vi "Begin.vi"(11 "Image Size":T1=enum."160x120") -> (0 "error out":errorcluster)   [LabVIEW 2012]
doc: "Called before other user functions, this VI is expected to open initial I/O refnums, load in file data, and do all program initialization. Notice that the <B>error out</B> terminal is simply used for data flow. Wiring it to other structures or subVIs ensures that this VI runs first."
uses:
  <vilib>/Rock Robotics/WPI/Camera/WPI_CameraImageSize.ctl
  <vilib>/Rock Robotics/WPI/DriverStation/WPI_DriverStationRobotMode2.ctl
  <vilib>/Rock Robotics/WPI/Joystick/WPI_JoystickDeviceEnum.ctl
  <vilib>/Rock Robotics/WPI/CAN/Jaguar/SubVIs/WPI_CANJaguar_ControlMode.ctl
  <vilib>/Rock Robotics/WPI/CAN/Jaguar/SubVIs/WPI_CANJaguar_SpeedReference.ctl
  <vilib>/Rock Robotics/WPI/CAN/Jaguar/SubVIs/WPI_CANJaguar_BrakeCoastMode.ctl
  <vilib>/Rock Robotics/WPI/CAN/Jaguar/SubVIs/WPI_CANJaguar_PositionReference.ctl
  <vilib>/Rock Robotics/SystemInterfaces/Typedef/FPGA_TypedefDigitalModule.ctl
  <vilib>/Rock Robotics/SystemInterfaces/DIO/FPGA_DIOChannel.ctl
  <vilib>/Rock Robotics/SystemInterfaces/DIO/FPGA_DIORelayChannel.ctl
  <vilib>/Rock Robotics/SystemInterfaces/Typedef/FPGA_TypedefSolenoidModule.ctl
  <vilib>/Rock Robotics/WPI/Solenoid/WPI_SolenoidChannel.ctl
  Robot Global Data.vi
  <vilib>/Rock Robotics/WPI/MotorControl/WPI_MotorControlOpenCANJaguar.vi
  <vilib>/Rock Robotics/WPI/Solenoid/WPI_SolenoidOpenSingle.vi
  <vilib>/Rock Robotics/WPI/Compressor/WPI_CompressorGetSetRefNum.vi
  <vilib>/Rock Robotics/WPI/Camera/WPI_CameraWhite Balance Values.ctl
  <vilib>/Rock Robotics/WPI/Camera/WPI_CameraExposure Values.ctl
  <vilib>/Rock Robotics/WPI/Camera/WPI_CameraFrameRate.ctl
  <vilib>/Rock Robotics/WPI/RobotDrive/WPI_RobotDriveOpen4MotorWithCANJaguar.vi
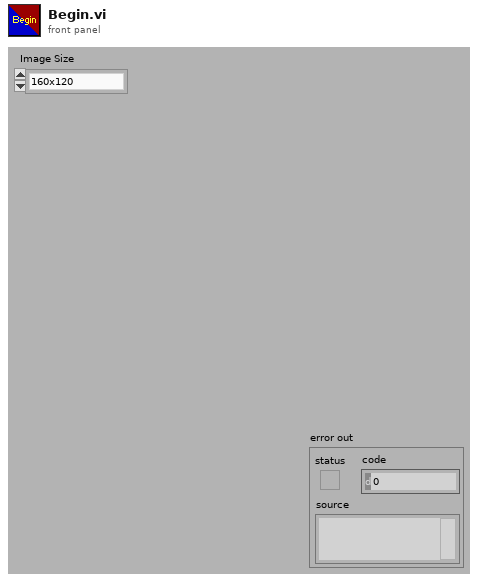
[diagram p1: front panel]
types:
  T1 = typedef "WPI_CameraImageSize.ctl" = enum16{"640x480", "320x240", "160x120"}
  T2 = typedef "WPI_SolenoidChannel.ctl" = enum8{"Solenoid 1", "Solenoid 2", "Solenoid 3", "Solenoid 4", "Solenoid 5", "Solenoid 6", "Solenoid 7", "Solenoid 8", "Invalid"}
  T3 = typedef "FPGA_TypedefSolenoidModule.ctl" = enum16{"Solenoid Module 1", "Solenoid Module 2"}
  T4 = typedef "FPGA_DIORelayChannel.ctl" = enum8{"Relay 1", "Relay 2", "Relay 3", "Relay 4", "Relay 5", "Relay 6", "Relay 7", "Relay 8", "Invalid"}
  T5 = typedef "FPGA_DIOChannel.ctl" = enum8{"DIO 1", "DIO 2", "DIO 3", "DIO 4", "DIO 5", "DIO 6", "DIO 7", "DIO 8", "DIO 9", "DIO 10", "DIO 11", "DIO 12", "DIO 13", "DIO 14", "Invalid"}
  T6 = typedef "FPGA_TypedefDigitalModule.ctl" = enum16{"Digital Module 1", "Digital Module 2"}
  T7 = typedef "WPI_JoystickDeviceEnum.ctl" = enum16{"USB 1", "USB 2", "USB 3", "USB 4", "Kinect 1", "Kinect 2"}
  T8 = typedef "WPI_CANJaguar_PositionReference.ctl" = u8
  T9 = typedef "WPI_CANJaguar_BrakeCoastMode.ctl" = enum8{"Jumper", "Brake", "Coast"}
  T10 = typedef "WPI_CANJaguar_ControlMode.ctl" = enum8{"Percent VBus", "Current", "Speed", "Position", "Voltage"}
  T11 = typedef "WPI_CANJaguar_SpeedReference.ctl" = u8
  T12 = typedef "WPI_DriverStationRobotMode2.ctl" = enum16{"Autonomous Disabled", "Autonomous Enabled", "Teleop Disabled", "Teleop Enabled", "Timeout", "Finish", "Test Disabled", "Test Enabled"}
  T13 = typedef "WPI_JoystickDevRef.ctl" = cluster{"Device":T7}
  T14 = typedef "WPI_DigitalInputDevRef.ctl" = cluster{"DevStatus":errorcluster, "DIO Channel":T5, "Digital Module":T6}
  T15 = typedef "WPI_CompressorDevRef.ctl" = cluster{"DevStatus":errorcluster, "DigitalInputDevRef":T14, "RelayDevRef":T16}
  T16 = typedef "WPI_RelayDevRef.ctl" = cluster{"DevStatus":errorcluster, "Relay Channel":T4, "Digital Module":T6, "Relay Direction":T17}
  T17 = typedef "WPI_RelayDirection.ctl" = enum16{"Both directions", "Forward only", "Reverse only"}
  T18 = typedef "WPI_SolenoidDevRef.ctl" = cluster{"DevStatus":errorcluster, "Solenoid Module":T3, "Forward Solenoid Channel":T2, "Reverse Solenoid Channel":T2}
  T19 = typedef "WPI_SerialPortRef.ctl" = cluster{"DevStatus":errorcluster, "Serial Port Name":refnum<visa-resource-name>}
  T20 = typedef "WPI_CameraFrameRate.ctl" = u32
  T21 = typedef "WPI_CameraExposure Values.ctl" = enum16{"Auto", "Flicker-free 50 Hz", "Flicker-free 60 Hz", "Hold current"}
  T22 = typedef "WPI_CameraWhite Balance Values.ctl" = enum16{"Auto", "Fixed indoor", "Fixed outdoor 1", "Fixed outdoor 2", "Fixed fluorescent 1", "Fixed fluorescent 2", "Hold current"}
  T23 = typedef "WPI_CameraDevRef.ctl" = cluster{"Camera Address":string, "CameraStatus":errorcluster, "Acquire Image Notifier":refnum<notifier>}
  T24 = typedef "WPI_MotorControlDeviceRef.ctl" = cluster{"DeviceStatus":errorcluster, "Type":enum16{"PWM", "CAN"}, "PWM":cluster{"Digital Module":T6, "PWM Channel":T25, "DeadBand":T26}, "CAN":cluster{"Device Number":u8, "Control Mode":T10, "Semaphore":T27, "Max Vout":dbl}, "Invert":bool, "TransformRef":T28, "InvTransformRef":T28}
  T25 = typedef "FPGA_DIOPWMChannel.ctl" = enum8{"PWM 1", "PWM 2", "PWM 3", "PWM 4", "PWM 5", "PWM 6", "PWM 7", "PWM 8", "PWM 9", "PWM 10", "Invalid"}
  T26 = typedef "WPI_PWMDeadband.ctl" = cluster{"Name":string, "maxPositivePwm":i32, "minPositivePwm":i32, "centerPwm":i32, "maxNegativePwm":i32, "minNegativePwm":i32, "angularRange":u16}
  T27 = typedef "Semaphore RefNum" = refnum<k1>
  T28 = typedef "WPI_PWMTransform_ConPane.ctl" = refnum<vi>
  T29 = typedef "WPI_RobotDriveDevRef.ctl" = cluster{"DevStatus":errorcluster, "Motors[]":T24[], "Square Inputs":bool, "Max Output":dbl, "Isochronous":bool}
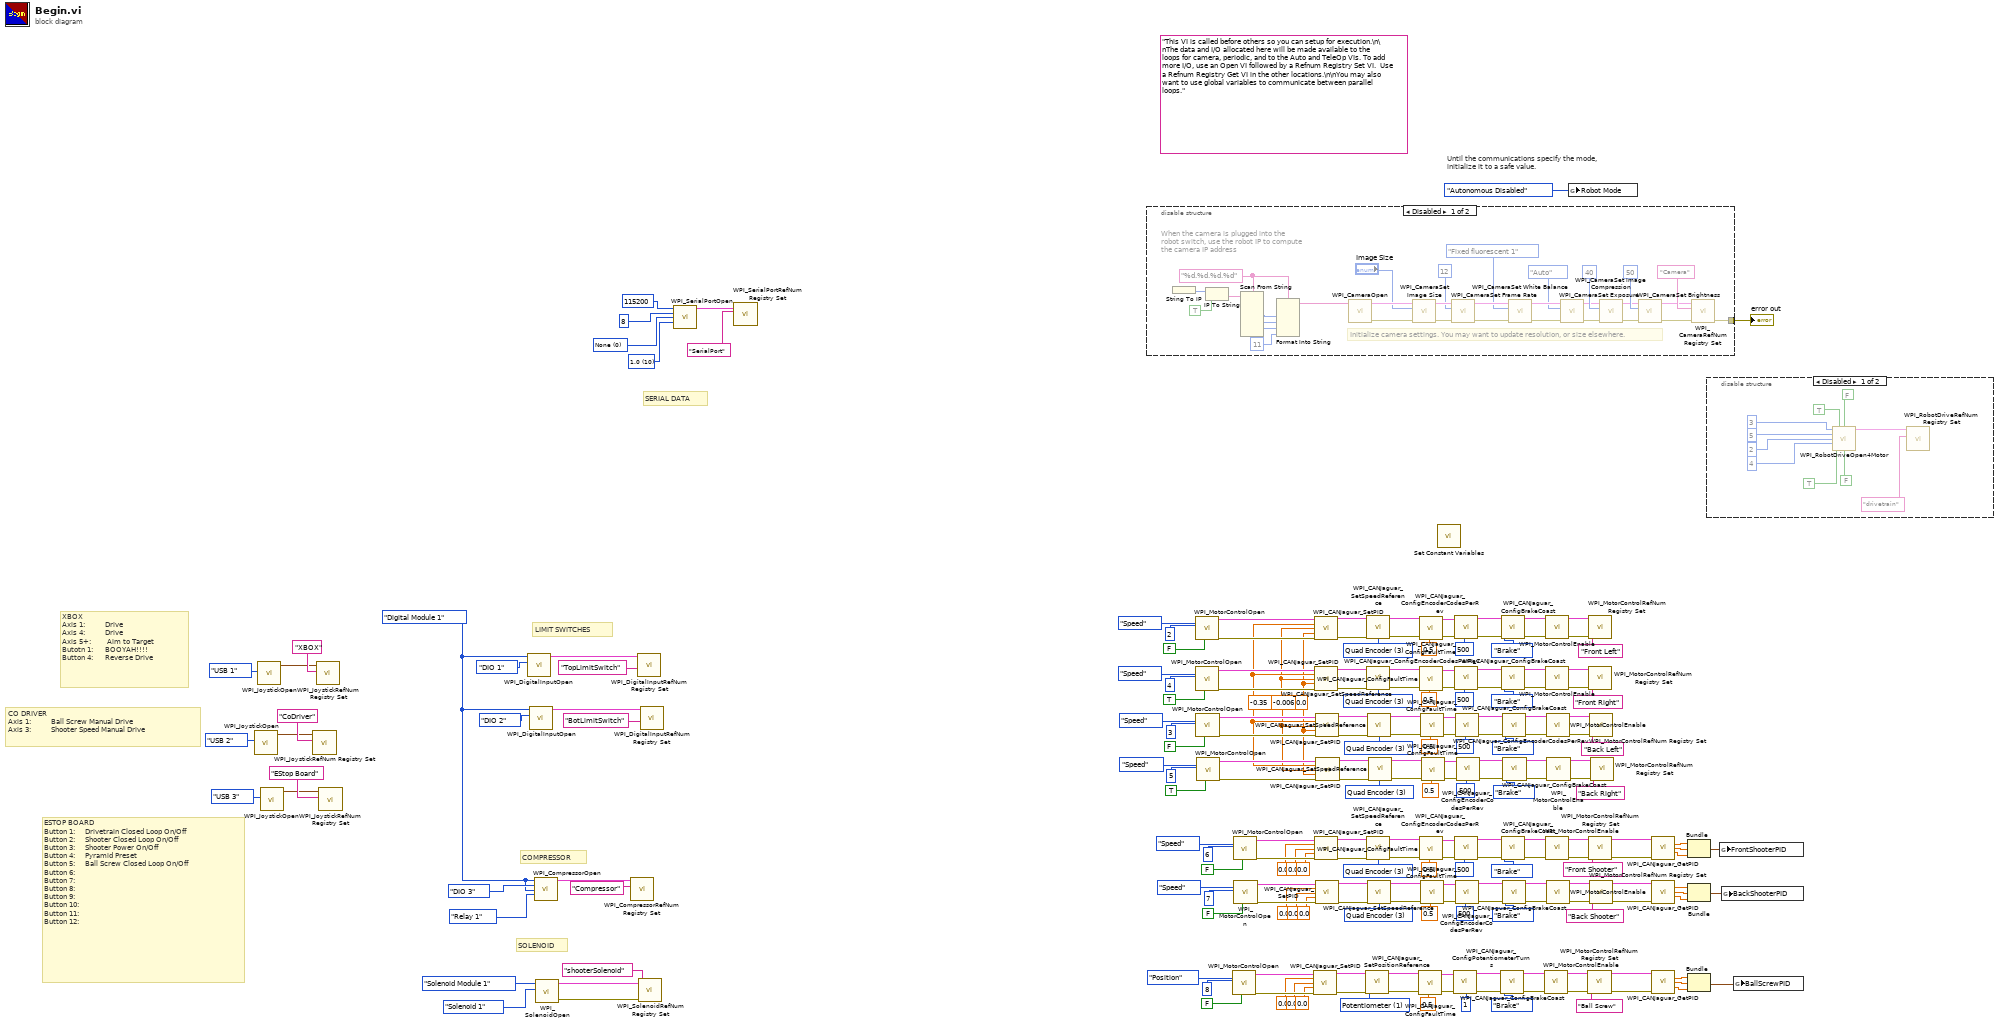
[diagram p0: block diagram]
diagram:
  w9 = FPGA_TypedefDigitalModule."Digital Module 1" ("Digital Module (Module 1)")
  w20 = -0.35 ("P")
  w19 = -0.006 ("I")
  w18 = 0.0 ("D")
  w45 = T8 1 items=["Quad Encoder"=0, "Potentiometer"=1, "None"=255] ("Position Reference")
  w83 = T11 3 items=["Encoder"=0, "Inv Encoder"=2, "Quad Encoder"=3, "None"=255] ("Speed Reference")
  w108 = T11 3 items=["Encoder"=0, "Inv Encoder"=2, "Quad Encoder"=3, "None"=255] ("Speed Reference")
  w130 = T11 3 items=["Encoder"=0, "Inv Encoder"=2, "Quad Encoder"=3, "None"=255] ("Speed Reference")
  w152 = T11 3 items=["Encoder"=0, "Inv Encoder"=2, "Quad Encoder"=3, "None"=255] ("Speed Reference")
  w174 = T11 3 items=["Encoder"=0, "Inv Encoder"=2, "Quad Encoder"=3, "None"=255] ("Speed Reference")
  w196 = T11 3 items=["Encoder"=0, "Inv Encoder"=2, "Quad Encoder"=3, "None"=255] ("Speed Reference")
  w209 = u16 10 items=["1.0"=10, "1.5"=15, "2.0"=20] ("Stop Bits")
  w210 = u16 0 items=["None", "Odd", "Even", "Mark", "Space"] ("Parity")
  (unwired) "This VI is called before others so you can setup for execution.\n\nThe data and I/O allocated here will be made available to the loops for camera, periodic, and to the Auto and TeleOp VIs. To add more I/O, use an Open VI followed by a Refnum Registry Set VI.  Use a Refnum Registry Get VI in the other locations.\n\nYou may also want to use global variables to communicate between parallel loops."
  # "SOLENOID"
  # "SERIAL DATA"
  # "LIMIT SWITCHES"
  # "COMPRESSOR"
  # "CO DRIVER\nAxis 1:          Ball Screw Manual Drive\nAxis 3:          Shooter Speed Manual Drive"
  # "XBOX\nAxis 1:          Drive\nAxis 4:          Drive\nAxis 5+:        Aim to Target\nButotn 1:      BOOYAH!!!!\nButton 4:      Reverse Drive"
  # "ESTOP BOARD\nButton 1:     Drivetrain Closed Loop On/Off\nButton 2:     Shooter Closed Loop On/Off\nButton 3:     Shooter Power On/Off\nButton 4:     Pyramid Preset\nButton 5:     Ball Screw Closed Loop On/Off\nButton 6:     \nButton 7:\nButton 8:\nButton 9:\nButton 10:\nButton 11:\nButton 12:"
  # "Until the communications specify the mode,\ninitialize it to a safe value."
  n1 = call <vilib>:"WPI_JoystickOpen.vi"("JoystickDevice"=WPI_JoystickDeviceEnum."USB 2") -> ("JoystickDevRef"=w25:T13)  [unwired: 10 in]
  n2 = call <vilib>:"WPI_JoystickOpen.vi"("JoystickDevice"=WPI_JoystickDeviceEnum."USB 1") -> ("JoystickDevRef"=w215:T13)  [unwired: 10 in]
  n3 = call <vilib>:"WPI_JoystickOpen.vi"("JoystickDevice"=WPI_JoystickDeviceEnum."USB 3") -> ("JoystickDevRef"=w22:T13)  [unwired: 10 in]
  n4 = call <vilib>:"WPI_JoystickRefNum Registry Set.vi"("refnum name"="CoDriver", "JoystickDevRef"=w25) -> ()  [unwired: 8 in, 2 out]
  n5 = call <vilib>:"WPI_JoystickRefNum Registry Set.vi"("refnum name"="XBOX", "JoystickDevRef"=w215) -> ()  [unwired: 8 in, 2 out]
  n6 = call <vilib>:"WPI_JoystickRefNum Registry Set.vi"("refnum name"="EStop Board", "JoystickDevRef"=w22) -> ()  [unwired: 8 in, 2 out]
  n7 = call <vilib>:"WPI_DigitalInputOpen.vi"("DIO Channel"=FPGA_DIOChannel."DIO 1", "Digital Module (Module 1)"=w9) -> ("DigitalInputDevRef"=w15:T14)  [unwired: 8 in, 1 out]
  n8 = call <vilib>:"WPI_DigitalInputOpen.vi"("DIO Channel"=FPGA_DIOChannel."DIO 2", "Digital Module (Module 1)"=w9) -> ("DigitalInputDevRef"=w12:T14)  [unwired: 8 in, 1 out]
  n9 = call <vilib>:"WPI_CompressorOpen.vi"("Pressure Switch Digital Module (Module 1)"=w9, "Pressure Switch DIO Channel"=FPGA_DIOChannel."DIO 3", "Relay Digital Module (Module 1)"=w9, "Relay Channel"=FPGA_DIORelayChannel."Relay 1") -> ("CompressorDevRef"=w7:T15)  [unwired: 10 in, 1 out]
  n10 = call-poly <vilib>:"WPI_SolenoidOpen.vi"("Solenoid Channel"=WPI_SolenoidChannel."Solenoid 1", "Solenoid Module (Module 1)"=FPGA_TypedefSolenoidModule."Solenoid Module 1") -> ("error out"=w2:errorcluster, "SolenoidDevRef"=w3:T18)  [unwired: 8 in]
  n11 = call <vilib>:"WPI_CompressorRefNum Registry Set.vi"("refnum name"="Compressor", "CompressorDevRef"=w7) -> ()  [unwired: 8 in, 2 out]
  n12 = call <vilib>:"WPI_DigitalInputRefNum Registry Set.vi"("refnum name"="TopLimitSwitch", "DigitalInputDevRef"=w15) -> ()  [unwired: 8 in, 2 out]
  n13 = call <vilib>:"WPI_SolenoidRefNum Registry Set.vi"("error in (no error)"=w2, "refnum name"="shooterSolenoid", "SolenoidDevRef"=w3) -> ()  [unwired: 7 in, 2 out]
  n14 = call <vilib>:"WPI_DigitalInputRefNum Registry Set.vi"("refnum name"="BotLimitSwitch", "DigitalInputDevRef"=w12) -> ()  [unwired: 8 in, 2 out]
  n15 = call <vilib>:"WPI_SerialPortOpen.vi"("Baud Rate"=u32 115200, "Data Bits"=u16 8, "Parity"=w210, "Stop Bits"=w209) -> ("SerialPortRef"=w208:T19)  [unwired: 10 in, 1 out]
  n16 = call <vilib>:"WPI_SerialPortRefNum Registry Set.vi"("refnum name"="SerialPort", "SerialPortRef"=w208) -> ()  [unwired: 8 in, 2 out]
  n17 = disable-structure shown="Disabled" {
    disable-tunnel: [w218 _] -> w213
    frame Disabled {
      w220 = "%d.%d.%d.%d" ("format string")
      # "When the camera is plugged into the\nrobot switch, use the robot IP to compute\nthe camera IP address"
      # "Initialize camera settings. You may want to update resolution, or size elsewhere."
      n18 = String To IP() -> (0:w227:u32)  [unwired: 1 in]
      n19 = IP To String(1:TRUE ("dot notation? (F)"), 2:w227) -> (0:w225:string)
      n20 = Scan From String(format string=w220, input string=w225) -> (output 1=w224:i32, output 2=w223:i32, output 3=w222:i32)  [unwired: 7 in, 3 out]
      n21 = Format Into String(format string=w220, w224, w223, w222, 11 ("Compression")) -> (resulting string=w219:string)  [unwired: 2 in, 1 out]
      n22 = call <vilib>:"WPI_CameraOpen.vi"("Camera Address"=w219) -> ("error out"=w239:errorcluster, "CameraDevRef"=w240:T23)  [unwired: 1 in, 8 out]
      n23 = call <vilib>:"WPI_CameraSet Image Size.vi"("error in (no error)"=w239, "Image Size"="Image Size", "CameraDevRef"=w240) -> ("error out"=w238:errorcluster, "CameraDevRef Out"=w241:T23)  [unwired: 7 out]
      n24 = call <vilib>:"WPI_CameraSet Frame Rate.vi"("error in (no error)"=w238, "Frame Rate (fps)"=T20 12, "CameraDevRef"=w241) -> ("error out"=w237:errorcluster, "CameraDevRef Out"=w243:T23)  [unwired: 7 out]
      n25 = call <vilib>:"WPI_CameraSet White Balance.vi"("error in (no error)"=w237, "White Balance"=WPI_CameraWhite_Balance_Values."Fixed fluorescent 1", "CameraDevRef"=w243) -> ("error out"=w236:errorcluster, "CameraDevRef Out"=w242:T23)  [unwired: 7 out]
      n26 = call <vilib>:"WPI_CameraSet Exposure.vi"("error in (no error)"=w236, "Exposure"=WPI_CameraExposure_Values."Auto", "CameraDevRef"=w242) -> ("error out"=w235:errorcluster, "CameraDevRef Out"=w245:T23)  [unwired: 7 out]
      n27 = call <vilib>:"WPI_CameraSet Image Compression.vi"("error in (no error)"=w235, "Compression"=40, "CameraDevRef"=w245) -> ("error out"=w234:errorcluster, "CameraDevRef Out"=w244:T23)  [unwired: 7 out]
      n28 = call <vilib>:"WPI_CameraSet Brightness.vi"("error in (no error)"=w234, "Brightness"=50, "CameraDevRef"=w244) -> ("error out"=w232:errorcluster, "CameraDevRef Out"=w233:T23)  [unwired: 7 out]
      n29 = call <vilib>:"WPI_CameraRefNum Registry Set.vi"("error in (no error)"=w232, "refnum name"="Camera", "CameraDevRef"=w233) -> ("error out"=w218:errorcluster)  [unwired: 8 out]
    }
    frame Enabled {
    }
  }
  "error out" <- w213
  n30 = call-poly <vilib>:"WPI_MotorControlOpen.vi"("Invert"=FALSE, "Device Number"=u8 2, "Control Mode"=WPI_CANJaguar_ControlMode."Speed") -> ("error out"=w200:errorcluster, "MotorControlDeviceRef"=w199:T24)  [unwired: 7 in]
  n31 = call-poly <vilib>:"WPI_MotorControlOpen.vi"("Invert"=TRUE, "Device Number"=u8 4, "Control Mode"=WPI_CANJaguar_ControlMode."Speed") -> ("error out"=w178:errorcluster, "MotorControlDeviceRef"=w177:T24)  [unwired: 7 in]
  n32 = call-poly <vilib>:"WPI_MotorControlOpen.vi"("Invert"=FALSE, "Device Number"=u8 3, "Control Mode"=WPI_CANJaguar_ControlMode."Speed") -> ("error out"=w156:errorcluster, "MotorControlDeviceRef"=w155:T24)  [unwired: 7 in]
  n33 = call-poly <vilib>:"WPI_MotorControlOpen.vi"("Invert"=TRUE, "Device Number"=u8 5, "Control Mode"=WPI_CANJaguar_ControlMode."Speed") -> ("error out"=w134:errorcluster, "MotorControlDeviceRef"=w133:T24)  [unwired: 7 in]
  n34 = call-poly <vilib>:"WPI_MotorControlOpen.vi"("Invert"=FALSE, "Device Number"=u8 8, "Control Mode"=WPI_CANJaguar_ControlMode."Position") -> ("error out"=w62:errorcluster, "MotorControlDeviceRef"=w61:T24)  [unwired: 7 in]
  n35 = call-poly <vilib>:"WPI_MotorControlOpen.vi"("Invert"=FALSE, "Device Number"=u8 6, "Control Mode"=WPI_CANJaguar_ControlMode."Speed") -> ("error out"=w112:errorcluster, "MotorControlDeviceRef"=w111:T24)  [unwired: 7 in]
  n36 = call-poly <vilib>:"WPI_MotorControlOpen.vi"("Invert"=FALSE, "Device Number"=u8 7, "Control Mode"=WPI_CANJaguar_ControlMode."Speed") -> ("error out"=w87:errorcluster, "MotorControlDeviceRef"=w86:T24)  [unwired: 7 in]
  n37 = call <vilib>:"WPI_CANJaguar_SetPID.vi"("CAN Jaguar Ref"=w61, "P"=0.0, "I"=0.0, "D"=0.0, "error in (no error)"=w62) -> ("CAN Jaguar Ref Out"=w68:T24, "error out"=w67:errorcluster)  [unwired: 9 in]
  n38 = call <vilib>:"WPI_CANJaguar_SetPID.vi"("CAN Jaguar Ref"=w199, "P"=w20, "I"=w19, "D"=w18, "error in (no error)"=w200) -> ("CAN Jaguar Ref Out"=w206:T24, "error out"=w205:errorcluster)  [unwired: 9 in]
  n39 = call <vilib>:"WPI_CANJaguar_SetPID.vi"("CAN Jaguar Ref"=w177, "P"=w20, "I"=w19, "D"=w18, "error in (no error)"=w178) -> ("CAN Jaguar Ref Out"=w184:T24, "error out"=w183:errorcluster)  [unwired: 9 in]
  n40 = call <vilib>:"WPI_CANJaguar_SetPID.vi"("CAN Jaguar Ref"=w111, "P"=0.0, "I"=0.0, "D"=0.0, "error in (no error)"=w112) -> ("CAN Jaguar Ref Out"=w118:T24, "error out"=w117:errorcluster)  [unwired: 9 in]
  n41 = call <vilib>:"WPI_CANJaguar_SetPID.vi"("CAN Jaguar Ref"=w155, "P"=w20, "I"=w19, "D"=w18, "error in (no error)"=w156) -> ("CAN Jaguar Ref Out"=w162:T24, "error out"=w161:errorcluster)  [unwired: 9 in]
  n42 = call <vilib>:"WPI_CANJaguar_SetPID.vi"("CAN Jaguar Ref"=w86, "P"=0.0, "I"=0.0, "D"=0.0, "error in (no error)"=w87) -> ("CAN Jaguar Ref Out"=w93:T24, "error out"=w92:errorcluster)  [unwired: 9 in]
  n43 = call <vilib>:"WPI_CANJaguar_SetPID.vi"("CAN Jaguar Ref"=w133, "P"=w20, "I"=w19, "D"=w18, "error in (no error)"=w134) -> ("CAN Jaguar Ref Out"=w140:T24, "error out"=w139:errorcluster)  [unwired: 9 in]
  n44 = call <vilib>:"WPI_CANJaguar_SetPositionReference.vi"("error in (no error)"=w67, "Position Reference"=w45, "CAN Jaguar Ref"=w68) -> ("error out"=w66:errorcluster, "CAN Jaguar Ref Out"=w65:T24)  [unwired: 7 in]
  n45 = call <vilib>:"WPI_CANJaguar_SetSpeedReference.vi"("error in (no error)"=w205, "Speed Reference"=w196, "CAN Jaguar Ref"=w206) -> ("error out"=w204:errorcluster, "CAN Jaguar Ref Out"=w203:T24)  [unwired: 7 in]
  n46 = call <vilib>:"WPI_CANJaguar_SetSpeedReference.vi"("error in (no error)"=w183, "Speed Reference"=w174, "CAN Jaguar Ref"=w184) -> ("error out"=w182:errorcluster, "CAN Jaguar Ref Out"=w181:T24)  [unwired: 7 in]
  n47 = call <vilib>:"WPI_CANJaguar_SetSpeedReference.vi"("error in (no error)"=w117, "Speed Reference"=w108, "CAN Jaguar Ref"=w118) -> ("error out"=w116:errorcluster, "CAN Jaguar Ref Out"=w115:T24)  [unwired: 7 in]
  n48 = call <vilib>:"WPI_CANJaguar_SetSpeedReference.vi"("error in (no error)"=w161, "Speed Reference"=w152, "CAN Jaguar Ref"=w162) -> ("error out"=w160:errorcluster, "CAN Jaguar Ref Out"=w159:T24)  [unwired: 7 in]
  n49 = call <vilib>:"WPI_CANJaguar_SetSpeedReference.vi"("error in (no error)"=w92, "Speed Reference"=w83, "CAN Jaguar Ref"=w93) -> ("error out"=w91:errorcluster, "CAN Jaguar Ref Out"=w90:T24)  [unwired: 7 in]
  n50 = call <vilib>:"WPI_CANJaguar_SetSpeedReference.vi"("error in (no error)"=w139, "Speed Reference"=w130, "CAN Jaguar Ref"=w140) -> ("error out"=w138:errorcluster, "CAN Jaguar Ref Out"=w137:T24)  [unwired: 7 in]
  n51 = call <vilib>:"WPI_CANJaguar_ConfigFaultTime.vi"("error in (no error)"=w66, "Fault Time (s)"=0.5, "CAN Jaguar Ref"=w65) -> ("error out"=w63:errorcluster, "CAN Jaguar Ref Out"=w64:T24)  [unwired: 7 in]
  n52 = call <vilib>:"WPI_CANJaguar_ConfigFaultTime.vi"("error in (no error)"=w204, "Fault Time (s)"=0.5, "CAN Jaguar Ref"=w203) -> ("error out"=w201:errorcluster, "CAN Jaguar Ref Out"=w202:T24)  [unwired: 7 in]
  n53 = call <vilib>:"WPI_CANJaguar_ConfigFaultTime.vi"("error in (no error)"=w182, "Fault Time (s)"=0.5, "CAN Jaguar Ref"=w181) -> ("error out"=w179:errorcluster, "CAN Jaguar Ref Out"=w180:T24)  [unwired: 7 in]
  n54 = call <vilib>:"WPI_CANJaguar_ConfigFaultTime.vi"("error in (no error)"=w116, "Fault Time (s)"=0.5, "CAN Jaguar Ref"=w115) -> ("error out"=w113:errorcluster, "CAN Jaguar Ref Out"=w114:T24)  [unwired: 7 in]
  n55 = call <vilib>:"WPI_CANJaguar_ConfigFaultTime.vi"("error in (no error)"=w160, "Fault Time (s)"=0.5, "CAN Jaguar Ref"=w159) -> ("error out"=w157:errorcluster, "CAN Jaguar Ref Out"=w158:T24)  [unwired: 7 in]
  n56 = call <vilib>:"WPI_CANJaguar_ConfigFaultTime.vi"("error in (no error)"=w91, "Fault Time (s)"=0.5, "CAN Jaguar Ref"=w90) -> ("error out"=w88:errorcluster, "CAN Jaguar Ref Out"=w89:T24)  [unwired: 7 in]
  n57 = call <vilib>:"WPI_CANJaguar_ConfigFaultTime.vi"("error in (no error)"=w138, "Fault Time (s)"=0.5, "CAN Jaguar Ref"=w137) -> ("error out"=w135:errorcluster, "CAN Jaguar Ref Out"=w136:T24)  [unwired: 7 in]
  n58 = call "Set Constant Variables.vi"() -> ()  [unwired: 12 in]
  n59 = call <vilib>:"WPI_CANJaguar_ConfigPotentiometerTurns.vi"("error in (no error)"=w63, "Potentiometer Turns"=u16 1 ("Encoder Codes Per Rev"), "CAN Jaguar Ref"=w64) -> ("error out"=w57:errorcluster, "CAN Jaguar Ref Out"=w56:T24)  [unwired: 7 in]
  n60 = call <vilib>:"WPI_CANJaguar_ConfigEncoderCodesPerRev.vi"("error in (no error)"=w201, "Encoder Codes Per Rev"=u16 500, "CAN Jaguar Ref"=w202) -> ("error out"=w193:errorcluster, "CAN Jaguar Ref Out"=w192:T24)  [unwired: 7 in]
  n61 = call <vilib>:"WPI_CANJaguar_ConfigEncoderCodesPerRev.vi"("error in (no error)"=w179, "Encoder Codes Per Rev"=u16 500, "CAN Jaguar Ref"=w180) -> ("error out"=w171:errorcluster, "CAN Jaguar Ref Out"=w170:T24)  [unwired: 7 in]
  n62 = call <vilib>:"WPI_CANJaguar_ConfigEncoderCodesPerRev.vi"("error in (no error)"=w113, "Encoder Codes Per Rev"=u16 500, "CAN Jaguar Ref"=w114) -> ("error out"=w105:errorcluster, "CAN Jaguar Ref Out"=w104:T24)  [unwired: 7 in]
  n63 = call <vilib>:"WPI_CANJaguar_ConfigEncoderCodesPerRev.vi"("error in (no error)"=w157, "Encoder Codes Per Rev"=u16 500, "CAN Jaguar Ref"=w158) -> ("error out"=w149:errorcluster, "CAN Jaguar Ref Out"=w148:T24)  [unwired: 7 in]
  n64 = call <vilib>:"WPI_CANJaguar_ConfigEncoderCodesPerRev.vi"("error in (no error)"=w88, "Encoder Codes Per Rev"=u16 500, "CAN Jaguar Ref"=w89) -> ("error out"=w80:errorcluster, "CAN Jaguar Ref Out"=w79:T24)  [unwired: 7 in]
  n65 = call <vilib>:"WPI_CANJaguar_ConfigEncoderCodesPerRev.vi"("error in (no error)"=w135, "Encoder Codes Per Rev"=u16 500, "CAN Jaguar Ref"=w136) -> ("error out"=w127:errorcluster, "CAN Jaguar Ref Out"=w126:T24)  [unwired: 7 in]
  n66 = call <vilib>:"WPI_CANJaguar_ConfigBrakeCoast.vi"("error in (no error)"=w57, "Brake / Coast Mode"=WPI_CANJaguar_BrakeCoastMode."Brake", "CAN Jaguar Ref"=w56) -> ("error out"=w48:errorcluster, "CAN Jaguar Ref Out"=w49:T24)  [unwired: 7 in]
  n67 = call <vilib>:"WPI_CANJaguar_ConfigBrakeCoast.vi"("error in (no error)"=w193, "Brake / Coast Mode"=WPI_CANJaguar_BrakeCoastMode."Brake", "CAN Jaguar Ref"=w192) -> ("error out"=w187:errorcluster, "CAN Jaguar Ref Out"=w188:T24)  [unwired: 7 in]
  n68 = call <vilib>:"WPI_CANJaguar_ConfigBrakeCoast.vi"("error in (no error)"=w171, "Brake / Coast Mode"=WPI_CANJaguar_BrakeCoastMode."Brake", "CAN Jaguar Ref"=w170) -> ("error out"=w165:errorcluster, "CAN Jaguar Ref Out"=w166:T24)  [unwired: 7 in]
  n69 = call <vilib>:"WPI_CANJaguar_ConfigBrakeCoast.vi"("error in (no error)"=w105, "Brake / Coast Mode"=WPI_CANJaguar_BrakeCoastMode."Brake", "CAN Jaguar Ref"=w104) -> ("error out"=w96:errorcluster, "CAN Jaguar Ref Out"=w97:T24)  [unwired: 7 in]
  n70 = call <vilib>:"WPI_CANJaguar_ConfigBrakeCoast.vi"("error in (no error)"=w149, "Brake / Coast Mode"=WPI_CANJaguar_BrakeCoastMode."Brake", "CAN Jaguar Ref"=w148) -> ("error out"=w143:errorcluster, "CAN Jaguar Ref Out"=w144:T24)  [unwired: 7 in]
  n71 = call <vilib>:"WPI_CANJaguar_ConfigBrakeCoast.vi"("error in (no error)"=w80, "Brake / Coast Mode"=WPI_CANJaguar_BrakeCoastMode."Brake", "CAN Jaguar Ref"=w79) -> ("error out"=w71:errorcluster, "CAN Jaguar Ref Out"=w72:T24)  [unwired: 7 in]
  n72 = call <vilib>:"WPI_CANJaguar_ConfigBrakeCoast.vi"("error in (no error)"=w127, "Brake / Coast Mode"=WPI_CANJaguar_BrakeCoastMode."Brake", "CAN Jaguar Ref"=w126) -> ("error out"=w121:errorcluster, "CAN Jaguar Ref Out"=w122:T24)  [unwired: 7 in]
  n73 = call <vilib>:"WPI_MotorControlEnable.vi"("error in (no error)"=w48, "CAN Jaguar Ref"=w49) -> ("error out"=w46:errorcluster, "CAN Jaguar Ref Out"=w47:T24)  [unwired: 8 in]
  n74 = call <vilib>:"WPI_MotorControlEnable.vi"("error in (no error)"=w187, "CAN Jaguar Ref"=w188) -> ("error out"=w185:errorcluster, "CAN Jaguar Ref Out"=w186:T24)  [unwired: 8 in]
  n75 = call <vilib>:"WPI_MotorControlEnable.vi"("error in (no error)"=w165, "CAN Jaguar Ref"=w166) -> ("error out"=w163:errorcluster, "CAN Jaguar Ref Out"=w164:T24)  [unwired: 8 in]
  n76 = call <vilib>:"WPI_MotorControlEnable.vi"("error in (no error)"=w96, "CAN Jaguar Ref"=w97) -> ("error out"=w94:errorcluster, "CAN Jaguar Ref Out"=w95:T24)  [unwired: 8 in]
  n77 = call <vilib>:"WPI_MotorControlEnable.vi"("error in (no error)"=w143, "CAN Jaguar Ref"=w144) -> ("error out"=w141:errorcluster, "CAN Jaguar Ref Out"=w142:T24)  [unwired: 8 in]
  n78 = call <vilib>:"WPI_MotorControlEnable.vi"("error in (no error)"=w71, "CAN Jaguar Ref"=w72) -> ("error out"=w69:errorcluster, "CAN Jaguar Ref Out"=w70:T24)  [unwired: 8 in]
  n79 = call <vilib>:"WPI_MotorControlEnable.vi"("error in (no error)"=w121, "CAN Jaguar Ref"=w122) -> ("error out"=w119:errorcluster, "CAN Jaguar Ref Out"=w120:T24)  [unwired: 8 in]
  n80 = global write "Robot Global Data.vi" "Robot Mode"(WPI_DriverStationRobotMode2."Autonomous Disabled" ("Robot Mode")) -> ()
  n81 = call <vilib>:"WPI_MotorControlRefNum Registry Set.vi"("error in (no error)"=w46, "refnum name"="Ball Screw", "MotorControlDevRef"=w47) -> ("error out"=w27:errorcluster, "MotorControlDevRef"=w28:T24)  [unwired: 7 in]
  n82 = call <vilib>:"WPI_MotorControlRefNum Registry Set.vi"("error in (no error)"=w185, "refnum name"="Front Left", "MotorControlDevRef"=w186) -> ()  [unwired: 7 in, 2 out]
  n83 = call <vilib>:"WPI_MotorControlRefNum Registry Set.vi"("error in (no error)"=w163, "refnum name"="Front Right", "MotorControlDevRef"=w164) -> ()  [unwired: 7 in, 2 out]
  n84 = call <vilib>:"WPI_MotorControlRefNum Registry Set.vi"("error in (no error)"=w94, "refnum name"="Front Shooter", "MotorControlDevRef"=w95) -> ("error out"=w31:errorcluster, "MotorControlDevRef"=w32:T24)  [unwired: 7 in]
  n85 = call <vilib>:"WPI_MotorControlRefNum Registry Set.vi"("error in (no error)"=w141, "refnum name"="Back Left", "MotorControlDevRef"=w142) -> ()  [unwired: 7 in, 2 out]
  n86 = call <vilib>:"WPI_MotorControlRefNum Registry Set.vi"("error in (no error)"=w69, "refnum name"="Back Shooter", "MotorControlDevRef"=w70) -> ("error out"=w29:errorcluster, "MotorControlDevRef"=w30:T24)  [unwired: 7 in]
  n87 = call <vilib>:"WPI_MotorControlRefNum Registry Set.vi"("error in (no error)"=w119, "refnum name"="Back Right", "MotorControlDevRef"=w120) -> ()  [unwired: 7 in, 2 out]
  n88 = call <vilib>:"WPI_CANJaguar_GetPID.vi"("CAN Jaguar Ref"=w32, "error in (no error)"=w31) -> ("P"=w43:dbl, "I"=w41:dbl, "D"=w42:dbl)  [unwired: 9 in, 2 out]
  n89 = call <vilib>:"WPI_CANJaguar_GetPID.vi"("CAN Jaguar Ref"=w30, "error in (no error)"=w29) -> ("P"=w39:dbl, "I"=w37:dbl, "D"=w38:dbl)  [unwired: 9 in, 2 out]
  n90 = call <vilib>:"WPI_CANJaguar_GetPID.vi"("CAN Jaguar Ref"=w28, "error in (no error)"=w27) -> ("P"=w35:dbl, "I"=w33:dbl, "D"=w34:dbl)  [unwired: 9 in, 2 out]
  n91 = Bundle("P"=w43, "I"=w41, "D"=w42) -> (w44:cluster{"P":dbl, "I":dbl, "D":dbl})  [unwired: 1 in]
  n92 = Bundle("P"=w39, "I"=w37, "D"=w38) -> (w40:cluster{"P":dbl, "I":dbl, "D":dbl})  [unwired: 1 in]
  n93 = Bundle("P"=w35, "I"=w33, "D"=w34) -> (w36:cluster{"P":dbl, "I":dbl, "D":dbl})  [unwired: 1 in]
  n94 = disable-structure shown="Disabled" {
    frame Disabled {
      n95 = call-poly <vilib>:"WPI_RobotDriveOpen4Motor.vi"("Rear Left Motor"=u8 3, "Rear Left Motor Inverted"=TRUE, "Rear Right Motor Inverted"=FALSE, "Rear Right Motor"=u8 5 ("Rear Left Motor"), "Front Left Motor"=u8 2 ("Rear Left Motor"), "Front Right Motor"=u8 4 ("Rear Left Motor"), "Front Left Motor Inverted"=TRUE, "Front Right Motor Inverted"=FALSE) -> ("RobotDriveDevRef"=w250:T29)  [unwired: 6 in, 1 out]
      n96 = call <vilib>:"WPI_RobotDriveRefNum Registry Set.vi"("refnum name"="drivetrain", "RobotDriveDevRef"=w250) -> ()  [unwired: 8 in, 2 out]
    }
    frame Enabled {
    }
  }
  n97 = global write "Robot Global Data.vi" "FrontShooterPID"(w44) -> ()
  n98 = global write "Robot Global Data.vi" "BackShooterPID"(w40) -> ()
  n99 = global write "Robot Global Data.vi" "BallScrewPID"(w36) -> ()
